vi "PI with FF_2.vi"(0 "Run PI?":bool, 1 "PIcluster":cluster{"SlewRate":dbl, "Kp":dbl, "Ki":dbl}, 2 "FFcluster":cluster{"FF_m":dbl, "FF_b":dbl}, 3 "LimitCluster":T1, 5 "SP":dbl, 7 "Error":dbl, 11 "RevCtrlZero":bool, 12 "IndirectMin?":bool, 13 "ApplySlew":bool, 14 "Indirect FF":bool) -> (4 "PreSlew":dbl, 8 "Output":dbl)   [LabVIEW 2013]
uses:
  <vilib>/addons/control/pid/pid.llb/PID Output Rate Limiter (DBL).vi
  <vilib>/addons/control/pid/NI_PID_pid.lvlib
panel:
  out "Step":dbl format="%.10g"
  out "slew output":dbl format="%.10f"
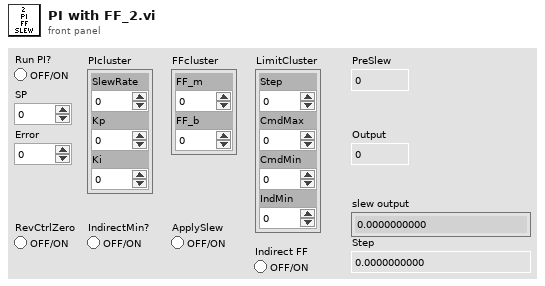
[diagram p1: front panel]
types:
  T1 = cluster{"Step":dbl, "CmdMax":dbl, "CmdMin":dbl, "IndMin":dbl}
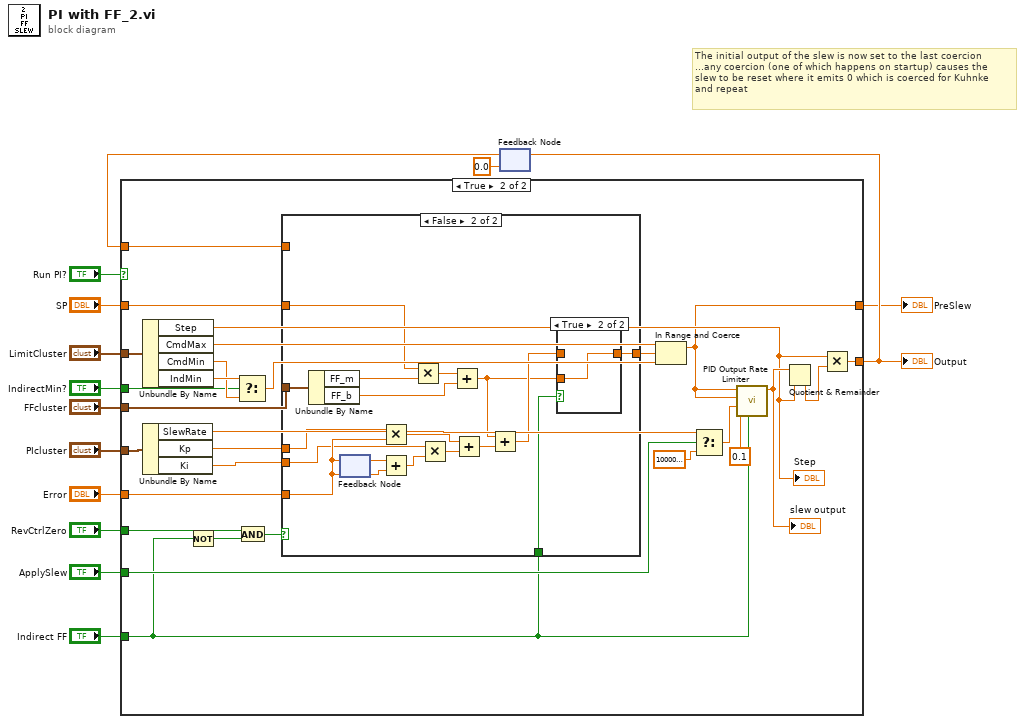
[diagram p0: block diagram]
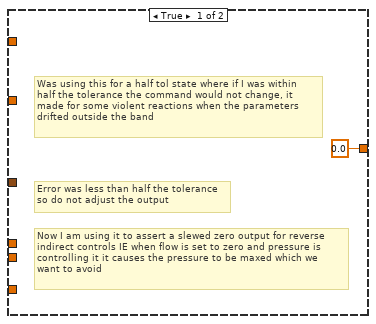
[diagram p3: hidden frame]
diagram:
  # "The initial output of the slew is now set to the last coercion\n...any coercion (one of which happens on startup) causes the\nslew to be reset where it emits 0 which is coerced for Kuhnke\nand repeat"
  n1 = feedback #1(0.0 ("SP")) -> (w13:dbl)
  n2 = case shown="True" "Run PI?" {
    tunnel: [w15 w32] -> w5
    tunnel: "SP" -> [w15 w43]
    tunnel: "Error" -> [_ w42]
    tunnel: "FFcluster" -> [_ w41]
    tunnel: "PIcluster" -> [_ w38]
    tunnel: "LimitCluster" -> [_ w39]
    tunnel: "RevCtrlZero" -> [_ w20]
    tunnel: w13 -> [_ w40]
    tunnel: "ApplySlew" -> [_ w17]
    tunnel: [w15 w18] -> w3
    tunnel: "IndirectMin?" -> [_ w22]
    tunnel: "Indirect FF" -> [_ w16]
    frame False {
    }
    frame True {
      n3 = Unbundle By Name(w39) -> ("Step"=w33:dbl, "CmdMax"=w30:dbl, "CmdMin"=w24:dbl, "IndMin"=w25:dbl)
      "Step" <- w33
      n4 = Unbundle By Name(w38) -> ("SlewRate"=w29:dbl, "Kp"=w37:dbl, "Ki"=w36:dbl)
      n5 = Not(x=w16) -> (.not. x?=w21:bool)
      n6 = Select(t=w25, s=w22, f=w24) -> (s? t:f=w23:dbl)
      n7 = And(x=w20, y=w21) -> (x .and. y?=w19:bool)
      n8 = case shown="False" w19 {
        tunnel: w43 -> [_ w59]
        tunnel: w42 -> [_ w57]
        tunnel: w41 -> [_ w53]
        tunnel: w40 -> [_ _]
        tunnel: w37 -> [_ w50]
        tunnel: w36 -> [_ w49]
        tunnel: [0.0 ("CmdMax") w47] -> w31
        tunnel: w16 -> [_ w45]
        frame True {
          # "Now I am using it to assert a slewed zero output for reverse\nindirect controls IE when flow is set to zero and pressure is\ncontrolling it it causes the pressure to be maxed which we\nwant to avoid"
          # "Was using this for a half tol state where if I was within\nhalf the tolerance the command would not change, it\nmade for some violent reactions when the parameters\ndrifted outside the band"
          # "Error was less than half the tolerance\nso do not adjust the output"
        }
        frame False {
          n9 = Unbundle By Name(w53) -> ("FF_m"=w52:dbl, "FF_b"=w51:dbl)
          n10 = feedback #2(w57) -> (w58:dbl)
          n11 = feedback-in #2(w57) -> ()
          n12 = Multiply(x=w50, y=w57) -> (x*y=w55:dbl)
          n13 = Add(x=w58, y=w57) -> (x+y=w54:dbl)
          n14 = Multiply(x=w59, y=w52) -> (x*y=w61:dbl)
          n15 = Multiply(x=w49, y=w54) -> (x*y=w56:dbl)
          n16 = Add(x=w61, y=w51) -> (x+y=w46:dbl)
          n17 = Add(x=w55, y=w56) -> (x+y=w60:dbl)
          n18 = Add(x=w46, y=w60) -> (x+y=w48:dbl)
          n19 = case shown="True" w45 {
            tunnel: w48 -> [w62 _]
            tunnel: [w62 w63] -> w47
            tunnel: w46 -> [_ w63]
            frame False {
            }
            frame True {
            }
          }
        }
      }
      n20 = In Range and Coerce(upper limit=w30, x=w31, lower limit=w23) -> (coerced(x)=w18:dbl)  [unwired: 1 out]
      n21 = Select(t=w29, s=w17, f=1000000.0) -> (s? t:f=w28:dbl)
      n22 = call-poly <vilib>:"PID Output Rate Limiter.vi"("reinitialize? (F)"=w16, "dt (s)"=0.1, "output rate (EGU/min)"=w28, "initial output"=w18, "input (controller output)"=w18) -> ("output"=w35:dbl)  [unwired: 3 in, 1 out]
      "slew output" <- w35
      n23 = Quotient & Remainder(x=w35, y=w33) -> (floor(x/y)=w34:dbl)  [unwired: 1 out]
      n24 = Multiply(x=w33, y=w34) -> (x*y=w32:dbl)
    }
  }
  "Output" <- w5
  "PreSlew" <- w3
  n25 = feedback-in #1(w5) -> ()
